vi "G#Object_GetEvent.vi"(1 "create if needed (T)":bool=TRUE, 2 "force create (F)":bool, 5 "error in (no error)":errorcluster) -> (15 "G# event":refnum<user-event>, 16 "created new":bool, 17 "valid":bool, 18 "event owner":string, 19 "error out":errorcluster)   [LabVIEW 2017, in "G#Object.lvclass"]
doc: "Returns the event used by the G#Object kernel to indicate that a new object has been created or has been deleted. This event is used by the debugger, but could be used by anyone."
uses:
  G#Object.lvclass
  utils/G#Object_Event.ctl
  utils/G#Object_EventType.ctl
  utils/G#Object_ObjectInfoType.ctl
  utils/G#Object_CreateMethod.ctl
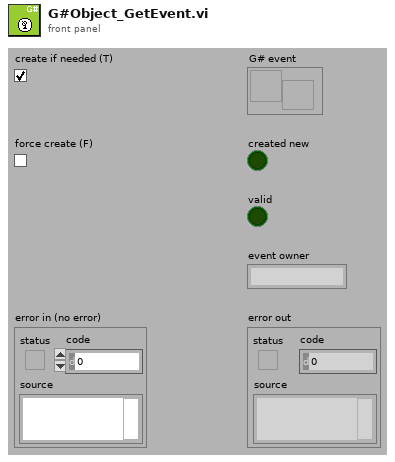
[diagram p1: front panel]
types:
  T1 = typedef "G#Object.lvclass/G#Object_Event.ctl" = cluster{"EventType":T2, "ObjectInfo":T3, "Ref":refnum<class "G#Object.lvclass">, "Time Stamp":timestamp, "LogText":string, "Parameters":variant[]}
  T2 = typedef "G#Object.lvclass/G#Object_EventType.ctl" = enum16{"Created new", "Looked up existing", "Deleted", "Forced delete", "Not deleted", "Garbage collected", "Cleared", "User", "Error", "External create object", "External create class attributes", "Created class attributes", "Run constructor", "Run constructor done", "Run open method", "Run open method done"}
  T3 = typedef "G#Object.lvclass/G#Object_ObjectInfoType.ctl" = cluster{"ObjectName":string, "ObjectID":u32, "Users":i32, "Counter":bool, "AttributeRefs":u32[], "FullClassName":string, "ClassName":string, "CreateMethod":T4, "GenericDestructorExists":bool, "Owner":string}
  T4 = typedef "G#Object.lvclass/G#Object_CreateMethod.ctl" = enum16{"Create", "Create or look up existing", "Look up existing"}
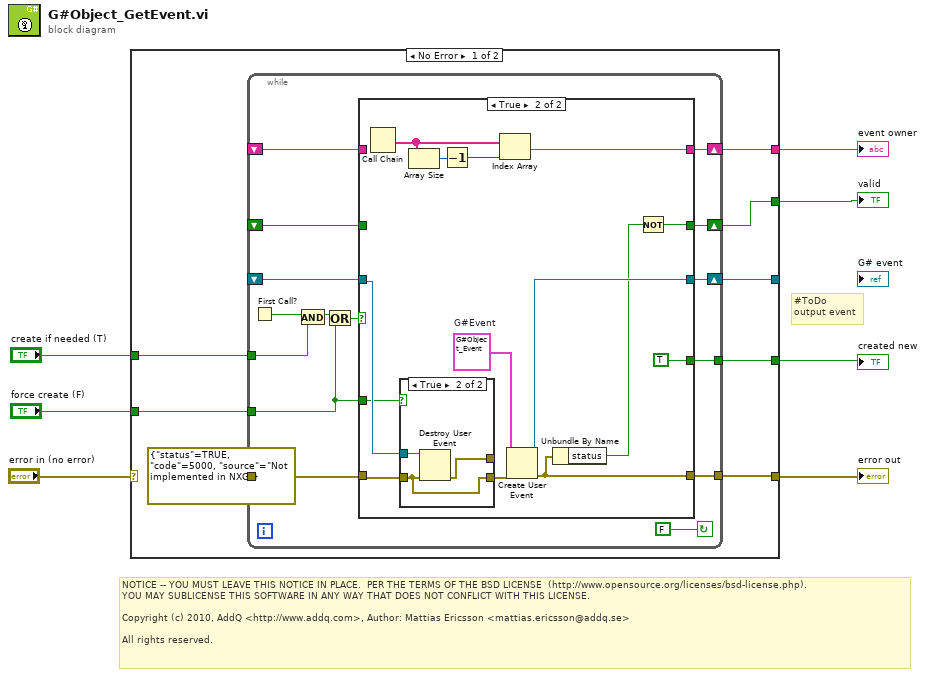
[diagram p0: block diagram]
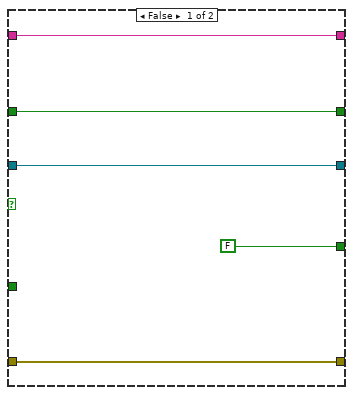
[diagram p2: hidden frame]
diagram:
  # "#ToDo\noutput event"
  # "NOTICE -- YOU MUST LEAVE THIS NOTICE IN PLACE.  PER THE TERMS OF THE BSD LICENSE  (http://www.opensource.org/licenses/bsd-license.php).\nYOU MAY SUBLICENSE THIS SOFTWARE IN ANY WAY THAT DOES NOT CONFLICT WITH THIS LICENSE.\n\nCopyright (c) 2010, AddQ <http://www.addq.com>, Author: Mattias Ericsson <mattias.ericsson@addq.se>\n\nAll rights reserved."
  n1 = case shown="No Error" "error in (no error)" {
    selector: "error in (no error)" -> [_ w54]
    tunnel: [w15 w54] -> w6
    tunnel: [w14 _] -> _
    tunnel: "create if needed (T)" -> [w13 _]
    tunnel: [w12 _] -> w3
    tunnel: [w11 _] -> w4
    tunnel: "force create (F)" -> [w10 _]
    tunnel: [w9 _] -> w1
    frame No Error {
      n2 = while {
        tunnel: errorcluster {"status"=TRUE, "code"=5000, "source"="Not implemented in NXG"} ("error out") -> [w29]
        shift-right: [w28] -> w14
        shift-left: _ -> [w26]
        tunnel: [w27] -> w15
        tunnel: w13 -> [w25]
        shift-right: [w24] -> w12
        shift-left: _ -> [w23]
        tunnel: [w22] -> w11
        tunnel: w10 -> [w18]
        shift-right: [w17] -> w9
        shift-left: _ -> [w16]
        stop <- FALSE continue-if-true
        n3 = First Call?() -> (First Call?: T/F=w19:bool)
        n4 = And(x=w19, y=w25) -> (x .and. y?=w20:bool)
        n5 = Or(x=w20, y=w18) -> (x .or. y?=w21:bool)
        n6 = case shown="True" w21 {
          tunnel: w29 -> [w34 w47]
          tunnel: [w35 w49] -> w28
          tunnel: [w34 w38] -> w27
          tunnel: w26 -> [w35 w45]
          tunnel: [w33 w41] -> w24
          tunnel: w23 -> [w33 _]
          tunnel: [FALSE TRUE] -> w22
          tunnel: w18 -> [_ w40]
          tunnel: [w31 w36] -> w17
          tunnel: w16 -> [w31 _]
          frame False {
          }
          frame True {
            w48 = T1 {"EventType"=enum."Created new", "ObjectInfo"={"ObjectName"="", "ObjectID"=0, "Users"=0, "Counter"=FALSE, "AttributeRefs"=[], "FullClassName"="", "ClassName"="", "CreateMethod"=enum."Create", "GenericDestructorExists"=FALSE, "Owner"=""}, "Ref"=refnum, "Time Stamp"=timestamp(0 s since 1904-01-01), "LogText"="", "Parameters"=[]}  # G#Event
            n7 = Call Chain() -> (call chain=w44:string[])
            n8 = case shown="True" w40 {
              tunnel: w47 -> [w50 w52]
              tunnel: [w50 w52] -> w46
              tunnel: w45 -> [_ w53]
              tunnel: [_ w51] -> _
              frame False {
              }
              frame True {
                n9 = Destroy User Event(user event=w53, error in=w52) -> (error out=w51:errorcluster)
              }
            }
            n10 = Array Size(array=w44) -> (size(s)=w43:i32)
            n11 = Decrement(x=w43) -> (x-1=w42:i32)
            n12 = Index Array(array=w44, index=w42) -> (element=w41:string)
            n13 = Create User Event(user event datatype=w48, error in=w46) -> (user event=w49:refnum<user-event>, error out=w38:errorcluster)
            n14 = Unbundle By Name(w38) -> ("status"=w37:bool)
            n15 = Not(x=w37) -> (.not. x?=w36:bool)
          }
        }
      }
    }
    frame Error {
    }
  }
  "error out" <- w6
  "valid" <- w1
  "created new" <- w4
  "event owner" <- w3
